vi "ALTS-2015 Read Test Data Result.vi"(8 "error in (no error)":errorcluster, 10 "Station Enum":T1, 11 "Status":enum16{"Pass", "Fail"}(ring)) -> (0 "error out":errorcluster, 3 "Same as Previous Test Result?":bool)   [LabVIEW 2013]
uses:
  Controls/ALTS-2015 Station Cluster.ctl
  Controls/ALTS-2015 Status Message Options.ctl
  Controls/ALTS-2015 Obtain Test Data DB Driver Options.ctl
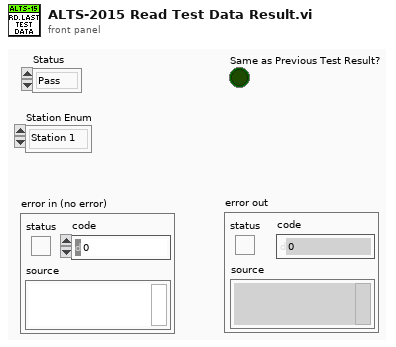
[diagram p1: front panel]
types:
  T1 = typedef "ALTS-2015 Station Cluster.ctl" = enum16{"Station 1", "Station 2", "Station 3", "Station 4"}
  T2 = typedef "ALTS-2015 Obtain Test Data DB Driver Options.ctl" = enum16{"Init", "Read Test Data Results", "Close"}
  T3 = typedef "ALTS-2015 Status Message Options.ctl" = enum16{"Initializing...", "Enter User Login...", "Enter Work Order Number...", "Enter Serial Number...", "Valid Serial Number...", "Invalid Serial Number...", "Start Tag Received...", "Stop Tag Received...", "UUT Clamped...", "UUT not Clamped...", "Test Running...", "Test Complete...", "Writing Result to DB...", "DB Entry Pressed...", "Clearing Serial Number...", "Idle...", "Exiting..."}
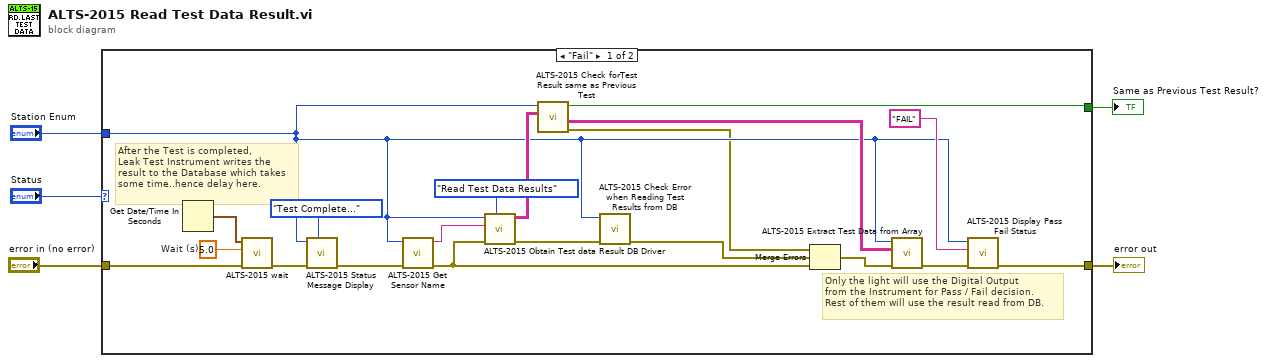
[diagram p0: block diagram]
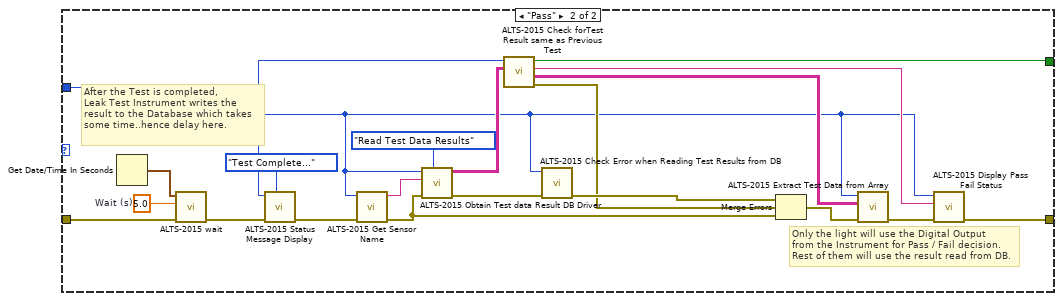
[diagram p2: hidden frame]
diagram:
  n1 = case shown="\"Fail\"" "Status" {
    tunnel: "Station Enum" -> [w7 w29]
    tunnel: "error in (no error)" -> [w8 w28]
    tunnel: [w10 w27] -> w3
    tunnel: [w9 w26] -> w1
    frame "Fail" {
      w15 = 5.0  # Wait (s)
      # "Only the light will use the Digital Output \nfrom the Instrument for Pass / Fail decision.\nRest of them will use the result read from DB."
      # "After the Test is completed, \nLeak Test Instrument writes the\nresult to the Database which takes\nsome time..hence delay here."
      n2 = Get Date/Time In Seconds() -> (seconds since 1Jan1904=w17:timestamp)
      n3 = call "ALTS-2015 wait.vi"("error in"=w8, "Wait (s)"=w15, "Start time"=w17) -> ("error out"=w16:errorcluster)  [unwired: 6 in, 2 out]
      n4 = call "ALTS-2015 Status Message Display.vi"("Status Message Options"=ALTS-2015_Status_Message_Options."Test Complete...", "error in (no error)"=w16, "Station Enum"=w7) -> ("error out"=w24:errorcluster)  [unwired: 7 in, 1 out]
      n5 = call "ALTS-2015 Get Sensor Name.vi"("error in (no error)"=w24, "Station Enum"=w7) -> ("error out"=w13:errorcluster, "Sensor Name"=w18:string)  [unwired: 8 in]
      n6 = call "ALTS-2015 Obtain Test data Result DB Driver.vi"("Option"=ALTS-2015_Obtain_Test_Data_DB_Driver_Options."Read Test Data Results", "error in"=w13, "Sensor Name"=w18, "Station Enum"=w7) -> ("error out"=w22:errorcluster, "data"=w12:string[][])  [unwired: 6 in]
      n7 = call "ALTS-2015 Check forTest Result same as Previous Test.vi"("Current Test Result"=w12, "Station Enum"=w7) -> ("error out"=w6:errorcluster, "Test Result"=w11:string[][], "Same as Previous Test Result?"=w9:bool)  [unwired: 6 in, 1 out]
      n8 = call "ALTS-2015 Check Error when Reading Test Results from DB.vi"("error in"=w22, "Station Enum"=w7) -> ("error out"=w19:errorcluster)  [unwired: 9 in]
      n9 = Merge Errors(w6, w19, w13) -> (w20:errorcluster)
      n10 = call "ALTS-2015 Extract Test Data from Array.vi"("error in"=w20, "data"=w11, "Station Enum"=w7) -> ("error out"=w23:errorcluster)  [unwired: 7 in, 1 out]
      n11 = call "ALTS-2015 Display Pass Fail Status.vi"("error in (no error)"=w23, "Test Result"="FAIL" ("y"), "Station Enum"=w7) -> ("error out"=w10:errorcluster)  [unwired: 8 in]
    }
    frame "Pass" {
      w36 = 5.0  # Wait (s)
      # "Only the light will use the Digital Output \nfrom the Instrument for Pass / Fail decision.\nRest of them will use the result read from DB."
      # "After the Test is completed, \nLeak Test Instrument writes the\nresult to the Database which takes\nsome time..hence delay here."
      n12 = Get Date/Time In Seconds() -> (seconds since 1Jan1904=w38:timestamp)
      n13 = call "ALTS-2015 wait.vi"("error in"=w28, "Wait (s)"=w36, "Start time"=w38) -> ("error out"=w37:errorcluster)  [unwired: 6 in, 2 out]
      n14 = call "ALTS-2015 Status Message Display.vi"("Status Message Options"=ALTS-2015_Status_Message_Options."Test Complete...", "error in (no error)"=w37, "Station Enum"=w29) -> ("error out"=w44:errorcluster)  [unwired: 7 in, 1 out]
      n15 = call "ALTS-2015 Get Sensor Name.vi"("error in (no error)"=w44, "Station Enum"=w29) -> ("error out"=w31:errorcluster, "Sensor Name"=w39:string)  [unwired: 8 in]
      n16 = call "ALTS-2015 Obtain Test data Result DB Driver.vi"("Option"=ALTS-2015_Obtain_Test_Data_DB_Driver_Options."Read Test Data Results", "error in"=w31, "Sensor Name"=w39, "Station Enum"=w29) -> ("error out"=w42:errorcluster, "data"=w33:string[][])  [unwired: 6 in]
      n17 = call "ALTS-2015 Check forTest Result same as Previous Test.vi"("Current Test Result"=w33, "Station Enum"=w29) -> ("error out"=w30:errorcluster, "Test Result"=w32:string[][], "Result Status"=w34:string, "Same as Previous Test Result?"=w26:bool)  [unwired: 6 in]
      n18 = call "ALTS-2015 Check Error when Reading Test Results from DB.vi"("error in"=w42, "Station Enum"=w29) -> ("error out"=w35:errorcluster)  [unwired: 9 in]
      n19 = Merge Errors(w35, w30, w31) -> (w40:errorcluster)
      n20 = call "ALTS-2015 Extract Test Data from Array.vi"("error in"=w40, "data"=w32, "Station Enum"=w29) -> ("error out"=w43:errorcluster)  [unwired: 7 in, 1 out]
      n21 = call "ALTS-2015 Display Pass Fail Status.vi"("error in (no error)"=w43, "Test Result"=w34, "Station Enum"=w29) -> ("error out"=w27:errorcluster)  [unwired: 8 in]
    }
  }
  "error out" <- w3
  "Same as Previous Test Result?" <- w1
